vi "Log Error and Build FGV.vi"(4 "Error Location":T1=enum."Compile HHP", 6 "Operation Mode":T2=enum."Open File", 8 "error in":errorcluster, 9 "Build Output":string, 10 "Log Build Output?":bool, 11 "Help Documentation Path":path) -> (0 "error out":errorcluster)   [LabVIEW 2016]
uses:
  Log FGV Operation Modes.ctl
  Error Location.ctl
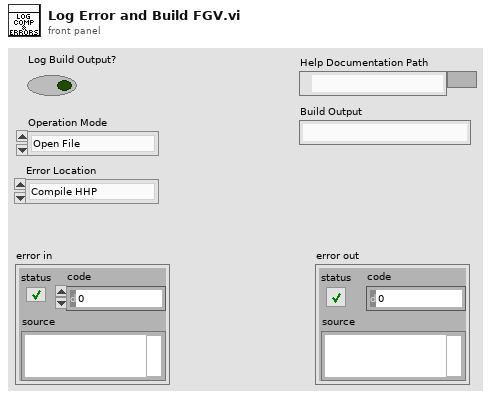
[diagram p1: front panel]
types:
  T1 = typedef "Error Location.ctl" = enum16{"Delete tmp", "Compile HHP", "Find Install", "Create tmp", "Create HHP", "Find Help"}
  T2 = typedef "Log FGV Operation Modes.ctl" = enum16{"Close", "Write", "Open File"}
  T3 = enum16{"open", "replace", "create", "open or create", "replace or create", "replace or create with confirmation"}
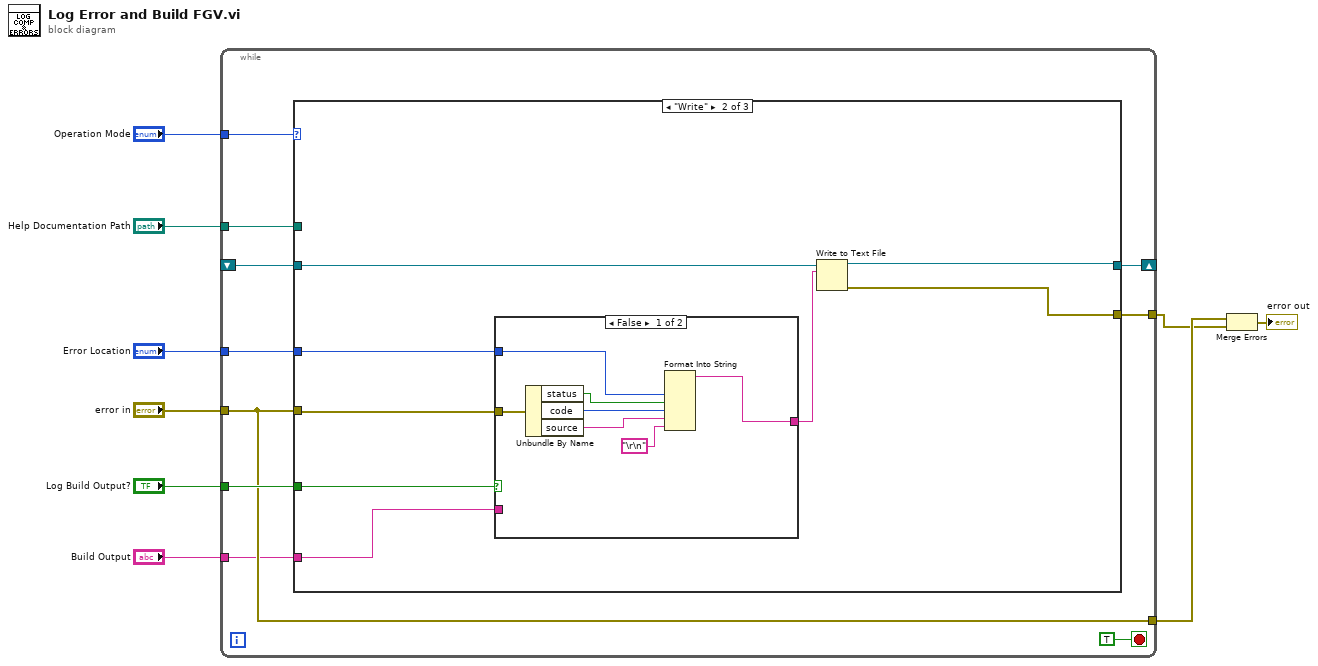
[diagram p0: block diagram]
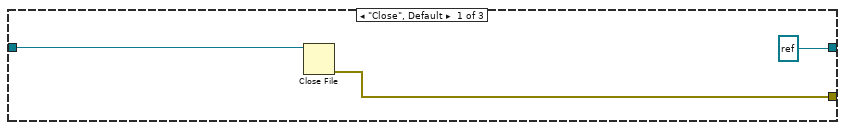
[diagram p2: hidden frame]
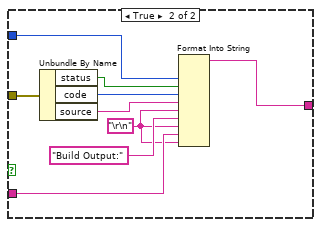
[diagram p3: hidden frame]
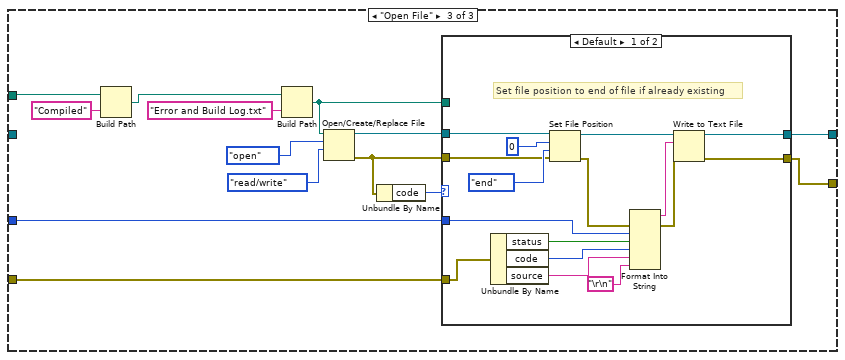
[diagram p4: hidden frame]
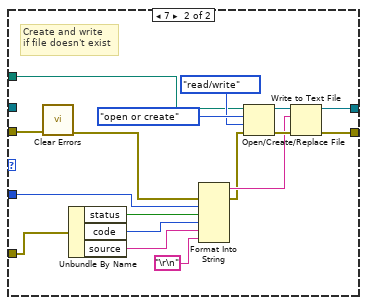
[diagram p5: hidden frame]
diagram:
  n1 = while {
    tunnel: "Operation Mode" -> [w18]
    shift-right: [w17] -> _
    shift-left: _ -> [w16]
    tunnel: "error in" -> [w12]
    tunnel: "Log Build Output?" -> [w15]
    tunnel: "Error Location" -> [w14]
    tunnel: [w13] -> w4
    tunnel: [w12] -> w5
    tunnel: "Build Output" -> [w11]
    tunnel: "Help Documentation Path" -> [w10]
    stop <- TRUE stop-if-true
    n2 = case shown="\"Write\"" w18 {
      tunnel: [w22 w28 w55] -> w13
      tunnel: [refnum<file> refnum ("refnum out") w29 w54] -> w17
      tunnel: w16 -> [w20 w30 _]
      tunnel: w12 -> [_ w27 w53]
      tunnel: w15 -> [_ w26 _]
      tunnel: w14 -> [_ w24 w52]
      tunnel: w11 -> [_ w23 _]
      tunnel: w10 -> [_ _ w49]
      frame "Close", Default {
        n3 = Close File(refnum=w20) -> (error out=w22:errorcluster)  [unwired: 1 in, 1 out]
      }
      frame "Write" {
        n4 = case shown="False" w26 {
          tunnel: w27 -> [w34 w43]
          tunnel: [w33 w42] -> w25
          tunnel: w24 -> [w32 w41]
          tunnel: w23 -> [_ w39]
          frame False {
            n5 = Unbundle By Name(w34) -> ("status"=w37:bool, "code"=w36:i32, "source"=w35:string)
            n6 = Format Into String(w32, w37, w36, w35, "\r\n") -> (resulting string=w33:string)  [unwired: 3 in, 1 out]
          }
          frame True {
            w38 = "\r\n"
            n7 = Unbundle By Name(w43) -> ("status"=w46:bool, "code"=w45:i32, "source"=w44:string)
            n8 = Format Into String(w41, w46, w45, w44, w38, "Build Output:" ("input 6"), w38, w39, w38) -> (resulting string=w42:string)  [unwired: 3 in, 1 out]
          }
        }
        n9 = Write to Text File(file (use dialog)=w30, text=w25) -> (refnum out=w29:refnum<file>, error out=w28:errorcluster)  [unwired: 2 in, 1 out]
      }
      frame "Open File" {
        n10 = Build Path(base path=w49, name or relative path="Compiled") -> (appended path=w47:path)
        n11 = Build Path(base path=w47, name or relative path="Error and Build Log.txt") -> (appended path=w50:path)
        n12 = Open/Create/Replace File(file path (use dialog)=w50, operation (0:open)=T3."open", access (0:read/write)=enum16{"read/write", "read-only", "write-only"}."read/write") -> (refnum out=w57:refnum<file>, error out=w56:errorcluster)  [unwired: 3 in, 1 out]
        n13 = Unbundle By Name(w56) -> ("code"=w58:i32)
        n14 = case shown="Default" w58 {
          tunnel: [w72 w88] -> w55
          tunnel: [w70 w89] -> w54
          tunnel: w57 -> [w74 _]
          tunnel: w56 -> [w73 w87]
          tunnel: w53 -> [w66 w81]
          tunnel: w52 -> [w65 w80]
          tunnel: w50 -> [_ w77]
          frame Default {
            # "Set file position to end of file if already existing"
            n15 = Unbundle By Name(w66) -> ("status"=w69:bool, "code"=w68:i32, "source"=w67:string)
            n16 = Set File Position(offset (in bytes) (0)=i64 0, refnum=w74, from (0:start)=enum16{"start", "end", "current"}."end", error in=w73) -> (refnum out=w71:refnum<file>, error out=w62:errorcluster)
            n17 = Format Into String(error in=w62, w65, w69, w68, w67, "\r\n") -> (resulting string=w64:string, error out=w61:errorcluster)  [unwired: 2 in]
            n18 = Write to Text File(file (use dialog)=w71, text=w64, error in=w61) -> (refnum out=w70:refnum<file>, error out=w72:errorcluster)  [unwired: 1 in, 1 out]
          }
          frame 7 {
            # "Create and write \nif file doesn't exist"
            n19 = call <vilib>:"Clear Errors.vi"("error in (no error)"=w87) -> ("error out"=w79:errorcluster)  [unwired: 5 in, 1 out]
            n20 = Unbundle By Name(w81) -> ("status"=w86:bool, "code"=w85:i32, "source"=w84:string)
            n21 = Format Into String(error in=w79, w80, w86, w85, w84, "\r\n") -> (resulting string=w82:string, error out=w78:errorcluster)  [unwired: 2 in]
            n22 = Open/Create/Replace File(file path (use dialog)=w77, error in=w78, operation (0:open)=T3."open or create", access (0:read/write)=enum16{"read/write", "read-only", "write-only"}."read/write") -> (refnum out=w91:refnum<file>, error out=w90:errorcluster)  [unwired: 2 in, 1 out]
            n23 = Write to Text File(file (use dialog)=w91, text=w82, error in=w90) -> (refnum out=w89:refnum<file>, error out=w88:errorcluster)  [unwired: 1 in, 1 out]
          }
        }
      }
    }
  }
  n24 = Merge Errors(w5, w4) -> (→"error out":errorcluster)
